vi "update_position.vi"(8 "error in (no error)":errorcluster, 11 "DL090409StageScaffold in":refnum<class "StageDL090409Scaffold.lvclass">) -> (0 "error out":errorcluster, 3 "DL090409StageScaffold out":refnum<class "StageDL090409Scaffold.lvclass">)   [LabVIEW 2010, in "StageDL090409Scaffold.lvclass"]
uses:
  StageDL090409Scaffold.lvclass
  StageDL090409Scaffold.lvclass/StageDL090409Scaffold.ctl
  common/classes/ErrorController/ErrorController/class_data.vi
  common/classes/SpaceVector/SpaceVector/SpaceVector.lvclass
  common/classes/ErrorController/ErrorController/ErrorController.lvclass
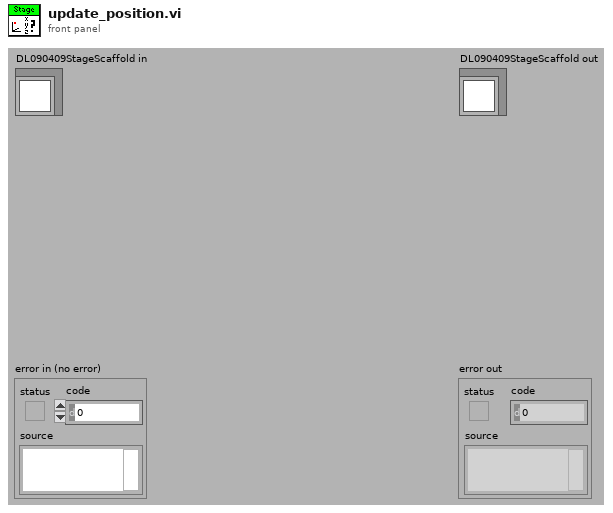
[diagram p1: front panel]
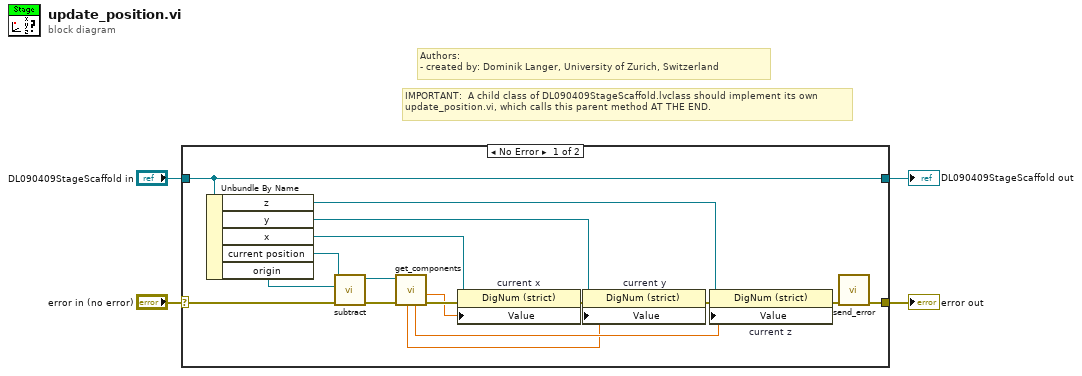
[diagram p0: block diagram]
diagram:
  # "IMPORTANT:  A child class of DL090409StageScaffold.lvclass should implement its own update_position.vi, which calls this parent method AT THE END."
  # "Authors: \n- created by: Dominik Langer, University of Zurich, Switzerland"
  n1 = case shown="No Error" "error in (no error)" {
    selector: "error in (no error)" -> [w9 w23]
    tunnel: [w10 w23] -> w3
    tunnel: [w21 w22] -> w1
    tunnel: "DL090409StageScaffold in" -> [w21 w22]
    frame No Error {
      n2 = Unbundle By Name(w21) -> ("z"=w12:refnum<vi>, "y"=w20:refnum<vi>, "x"=w13:refnum<vi>, "current position"=w7:refnum<class "SpaceVector.lvclass">, "origin"=w6:refnum<class "SpaceVector.lvclass">)
      n3 = call "subtract.vi"("error in (no error)"=w9, "subtrahend"=w6, "SpaceVector in"=w7) -> ("error out"=w8:errorcluster, "SpaceVector out"=w5:refnum<class "SpaceVector.lvclass">)  [unwired: 7 in]
      n4 = call "get_components.vi"("error in (no error)"=w8, "SpaceVector in"=w5) -> ("error out"=w17:errorcluster, "x"=w16:dbl[unit], "z"=w15:dbl[unit], "y"=w14:dbl[unit])  [unwired: 6 out]
      n5 = property on="current x" class="DigNum (strict)"(reference=w13, error in=w17, "Value"=w16) -> (error out=w19:errorcluster)  [unwired: 1 out]
      n6 = property on="current y" class="DigNum (strict)"(reference=w20, error in=w19, "Value"=w14) -> (error out=w18:errorcluster)  [unwired: 1 out]
      n7 = property on="current z" class="DigNum (strict)"(reference=w12, error in=w18, "Value"=w15) -> (error out=w11:errorcluster)  [unwired: 1 out]
      n8 = call "send_error.vi"("error in (no error)"=w11) -> ("error out"=w10:errorcluster)  [unwired: 10 in]
    }
    frame Error {
    }
  }
  "error out" <- w3
  "DL090409StageScaffold out" <- w1
